vi "event.create_programmatic.from_assets.vi"(4 "Additional Information":T1, 5 "Duration (0s)":dbl, 6 "Properties and Labels":T2, 7 "Time Stamp (now: system time)":timestamp format="%<%x %.3X>T", 8 "error in":errorcluster, 9 "Name":string, 10 "Asset RIDs":string[](array[string]), 11 "Nominal Client in":refnum<class "Nominal Client.lvclass">) -> (0 "error out":errorcluster, 3 "Nominal Client out":refnum<class "Nominal Client.lvclass">)   [LabVIEW 2020, in "Nominal Client.lvclass"]
doc: "Creates a timestamped event in Nominal associated with one or more assets, marking significant occurrences during test execution such as hardware state changes or sequence transitions. Events appear alongside telemetry data to enable correlation between test activities and system behavior during analysis."
uses:
  Nominal Client.lvclass
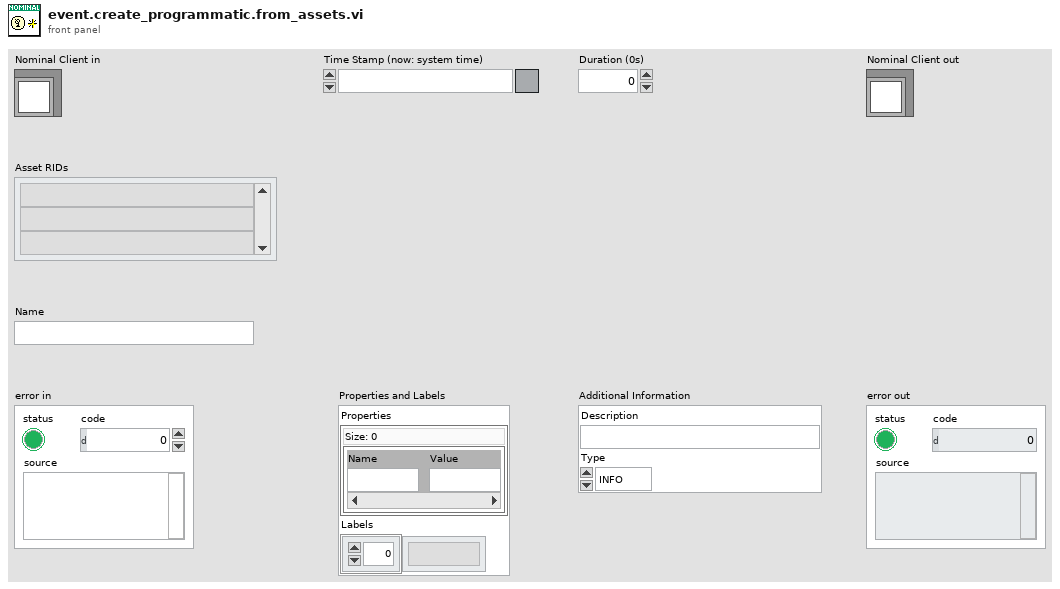
[diagram p1: front panel]
types:
  T1 = cluster{"Description":string, "Type":enum16{"INFO", "FLAG", "ERROR", "SUCCESS"}}
  T2 = cluster{"Properties":map{string, string}, "Labels":string[]}
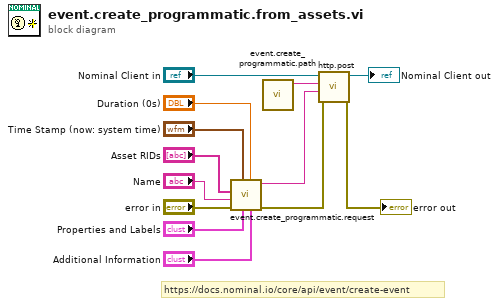
[diagram p0: block diagram]
diagram:
  # "https://docs.nominal.io/core/api/event/create-event"
  n1 = call "event.create_programmatic.request.vi"("Additional Information"="Additional Information", "Duration (0s)"="Duration (0s)", "Properties and Labels"="Properties and Labels", "Time Stamp (now: system time)"="Time Stamp (now: system time)", "error in"="error in", "Name"="Name", "Asset RIDs"="Asset RIDs") -> ("error out"=w3:errorcluster, "request"=w4:string)  [unwired: 3 in]
  n2 = call "event.create_programmatic.path.vi"() -> ("path"=w10:string)  [unwired: 11 in]
  n3 = call "http.post.vi"("error in"=w3, "Request body"=w4, "Path"=w10, "Nominal Client in"="Nominal Client in") -> ("error out"=→"error out":errorcluster, "Nominal Client out"=→"Nominal Client out":refnum<class "Nominal Client.lvclass">)  [unwired: 4 in, 2 out]
